vi "PenSolen.vi"(8 "error in (no error)":errorcluster caption="错误输入（无错误）", 10 "Bool引用":refnum<vi>, 11 "模式":enum16{"气缸向下", "气缸向上"}(ring)) -> (0 "error out":errorcluster caption="错误输出")   [LabVIEW 2011]
uses:
  <vilib>/Utility/error.llb/DialogType.ctl
  API/API DYM.lvlib
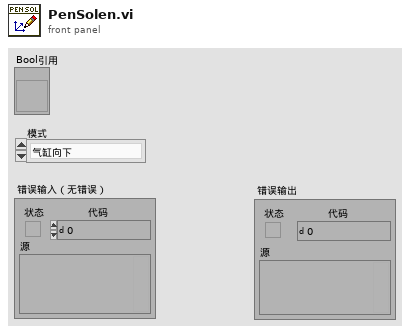
[diagram p1: front panel]
types:
  T1 = typedef "DialogType.ctl" = u16
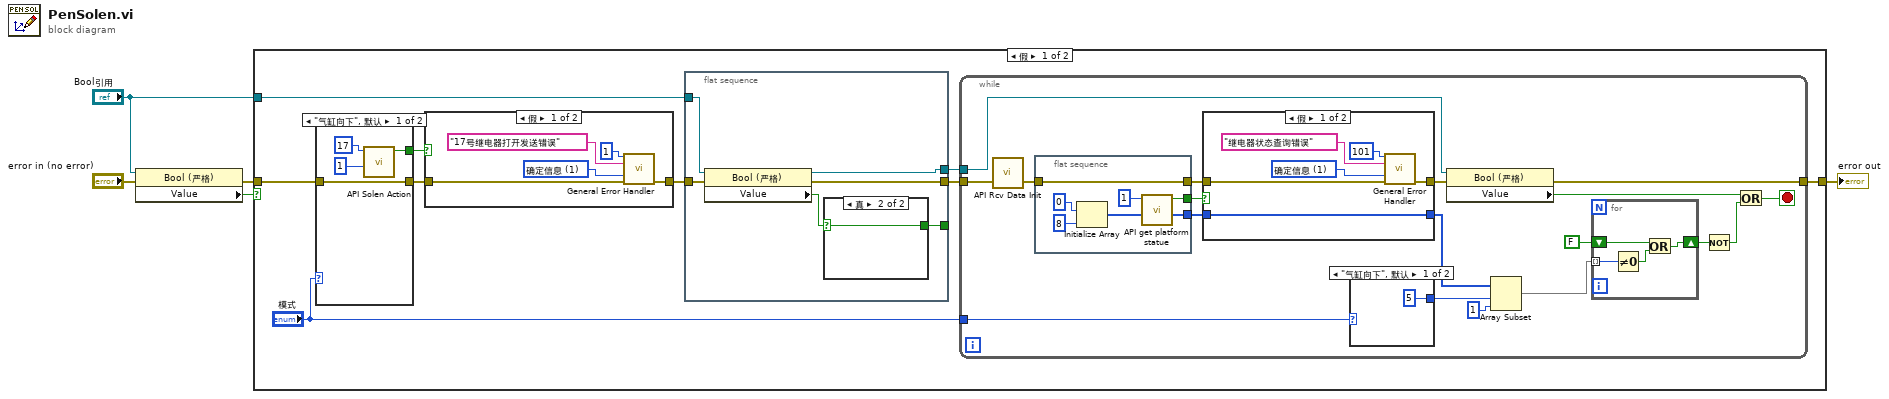
[diagram p0: block diagram]
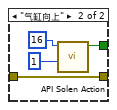
[diagram p2: hidden frame]
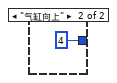
[diagram p3: hidden frame]
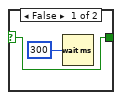
[diagram p5: hidden frame]
diagram:
  n1 = property on="属性节点" class="Bool (严格)"(reference="Bool引用", error in="error in (no error)") -> (error out=w3:errorcluster, "Value"=w4:bool)  [unwired: 1 out]
  n2 = case shown="假" w4 {
    tunnel: w3 -> [w6 w77]
    tunnel: "Bool引用" -> [w12 _]
    tunnel: [w9 w77] -> w1
    frame False {
      n3 = case shown="\"气缸向下\", 默认" "模式" {
        tunnel: [w16 w20] -> w14
        tunnel: w6 -> [w15 w19]
        tunnel: [w15 w19] -> w8
        frame "气缸向下", Default {
          n4 = call "API Solen Action.vi"("statue"=1, "solenNum"=17) -> ("solenaction return value"=w16:bool)  [unwired: 9 in]
        }
        frame "气缸向上" {
          n5 = call "API Solen Action.vi"("statue"=1, "solenNum"=16) -> ("solenaction return value"=w20:bool)  [unwired: 9 in]
        }
      }
      n6 = case shown="假" w14 {
        tunnel: w8 -> [w75 w76]
        tunnel: [w71 w76] -> w13
        frame False {
          w74 = T1 1 items=["无对话框", "确定信息", "继续或停止信息", "确定信息＋警告", "继续/停止+警告"] ("type of dialog (OK msg:1)")
          n7 = call <vilib>:"General Error Handler.vi"("[error code] (0)"=1, "[error source] (\" \")"="17号继电器打开发送错误" ("[error source] (\" \")"), "type of dialog (OK msg:1)"=w74, "error in (no error)"=w75) -> ("error out"=w71:errorcluster)  [unwired: 7 in, 4 out]
        }
        frame True {
        }
      }
      n8 = flat-sequence {
        tunnel: w13 -> [w65]
        tunnel: w12 -> [w67]
        tunnel: [w64] -> w11
        tunnel: [w63] -> _
        tunnel: [w62] -> w10
        frame #0 {
          n9 = property class="Bool (严格)"(reference=w67, error in=w65) -> (reference out=w62:refnum<vi>, error out=w64:errorcluster, "Value"=w66:bool)
          n10 = case shown="真" w66 {
            selector: w66 -> [w68 w70]
            tunnel: [w68 w70] -> w63
            frame False {
              n11 = Wait (ms)(milliseconds to wait=u32 300 ("等待时间（毫秒）")) -> ()  [unwired: 1 out]
            }
            frame True {
            }
          }
        }
      }
      n12 = while {
        tunnel: w11 -> [w25]
        tunnel: w10 -> [w38]
        tunnel: [w29] -> w9
        tunnel: "模式" -> [w28]
        stop <- w31 stop-if-true
        n13 = call "API Rcv Data Init.vi"("错误输入（无错误）"=w25) -> ("错误输出"=w24:errorcluster)  [unwired: 1 in, 1 out]
        n14 = flat-sequence {
          tunnel: [w43] -> w40
          tunnel: [w42] -> w39
          tunnel: w24 -> [w41]
          tunnel: [w41] -> w23
          frame #0 {
            n15 = Initialize Array(0, 8 ("维数大小")) -> (w44:i32[])
            n16 = call "API get platform statue.vi"("platformStatue input"=w44, "PlatformNum"=1) -> ("platformStatue output"=w42:i32[], "platformstatue return value"=w43:bool)  [unwired: 8 in]
          }
        }
        n17 = case shown="假" w40 {
          tunnel: w39 -> [w55 w61]
          tunnel: [w56 w60] -> w30
          tunnel: [w55 w61] -> w37
          tunnel: w23 -> [w54 w60]
          frame False {
            w57 = T1 1 items=["无对话框", "确定信息", "继续或停止信息", "确定信息＋警告", "继续/停止+警告"] ("type of dialog (OK msg:1)")
            n18 = call <vilib>:"General Error Handler.vi"("[error code] (0)"=101, "[error source] (\" \")"="继电器状态查询错误" ("[error source] (\" \")"), "type of dialog (OK msg:1)"=w57, "error in (no error)"=w54) -> ("error out"=w56:errorcluster)  [unwired: 7 in, 4 out]
          }
          frame True {
          }
        }
        n19 = case shown="\"气缸向下\", 默认" w28 {
          tunnel: [5 ("索引") 4 ("索引")] -> w27
          frame "气缸向下", Default {
          }
          frame "气缸向上" {
          }
        }
        n20 = property class="Bool (严格)"(reference=w38, error in=w30) -> (error out=w29:errorcluster, "Value"=w32:bool)  [unwired: 1 out]
        n21 = Array Subset(array=w37, index=w27, length=1 ("长度")) -> (w35:i32[])
        n22 = for {
          shift-right: [w51] -> w33
          shift-left: FALSE -> [w52]
          tunnel: w35 -> [w50] mode=indexing
          n23 = Not Equal To 0?(x=w50) -> (x != 0?=w53:bool)
          n24 = Or(x=w52, y=w53) -> (x .or. y?=w51:bool)
        }
        n25 = Not(x=w33) -> (.not. x?=w34:bool)
        n26 = Or(x=w32, y=w34) -> (x .or. y?=w31:bool)
      }
    }
    frame True {
    }
  }
  "error out" <- w1
